vi "Calculate # of Variables per Test.vi"(7 "Seq Parameters":T1={"Test Name"="Unique Test Name", "Target"=enum."cRIO-9012", "Host IP Address"="0.0.0.0", "Target IP Address"="0.0.0.0", "Shared Variable Host"=enum."Target", "Shared Variable Writer"=enum."Target", "Variable Data Type"=enum."Double", "# of Variables per Library"=500, "Update Rate (Hz)"=1.0, "Read Rate (Hz)"=1.0, "Floor"=500, "Ceiling"=5000, "Delta"=500} {"# of Variables per Library" items=["50"=50, "100"=100, "150"=150, "200"=200, "250"=250, "300"=300, "350"=350, "400"=400, "450"=450, "500"=500]; "Delta" min=50 max=1000000 step=50; "Ceiling" min=50 max=1000000 step=50; "Floor" min=50 max=1000000 step=50}, 8 "error in (no error)":errorcluster) -> (0 "error out":errorcluster, 3 "# of Variables per Test":u32[](array[numeric]))   [LabVIEW 2015]
doc: "Create an array that identifies the number of variables needed for each test in the sequence."
uses:
  Type Defs/Sequence Parameters.ctl
  Type Defs/Target Type.ctl
  Type Defs/Variable Data Type.ctl
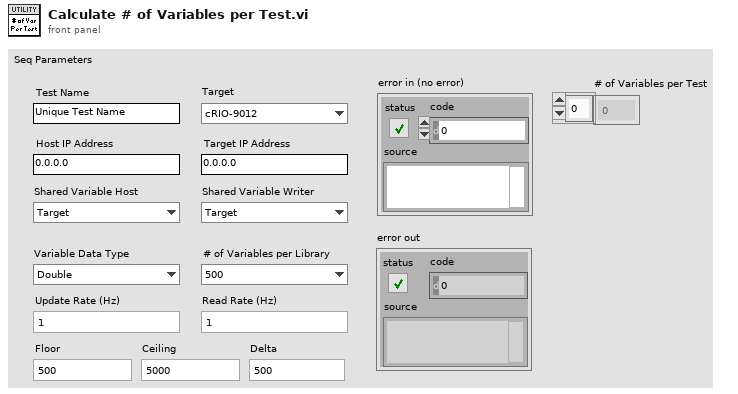
[diagram p1: front panel]
types:
  T1 = typedef "Sequence Parameters.ctl" = cluster{"Test Name":string, "Target":T2, "Host IP Address":string, "Target IP Address":string, "Shared Variable Host":enum16{"Target", "Host"}, "Shared Variable Writer":enum16{"Target", "Host"}, "Variable Data Type":T3, "# of Variables per Library":u16, "Update Rate (Hz)":dbl, "Read Rate (Hz)":dbl, "Floor":u32, "Ceiling":u32, "Delta":u32}
  T2 = typedef "Target Type.ctl" = enum16{"cRIO-9012", "cRIO-9014", "cRIO-9022", "cRIO-9023", "cRIO-9024", "cRIO-9025", "cRIO-9068", "cRIO-9073", "cRIO-9074", "cRIO-9075", "cRIO-9076", "cRIO-9081", "cRIO-9082", "myRIO-1900", "myRIO-1950", "PXI-8101", "PXI-8115", "PXI-8119", "PXI-8820", "PXIe-8100", "PXIe-8101", "PXIe-8133", "PXIe-8135", "PXIe-8820", "sbRIO-9605", "sbRIO-9606", "sbRIO-9623", "sbRIO-9626", "sbRIO-9633", "sbRIO-9636", "Unlisted (Linux-RT)", "Unlisted (PharLap)", "Unlisted (VxWorks)", "Windows Target"}
  T3 = typedef "Variable Data Type.ctl" = enum16{"U8", "U16", "U32", "U64", "I8", "I16", "I32", "I64", "Single", "Double", "Boolean", "String"}
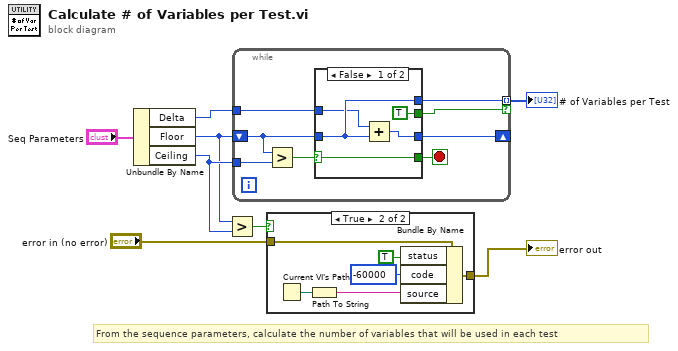
[diagram p0: block diagram]
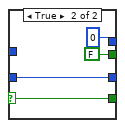
[diagram p3: hidden frame]
diagram:
  # "From the sequence parameters, calculate the number of variables that will be used in each test"
  n1 = Unbundle By Name("Seq Parameters") -> ("Delta"=w7:u32, "Floor"=w4:u32, "Ceiling"=w5:u32)
  n2 = Greater?(x=w4, y=w5) -> (0:w3:bool)
  n3 = while {
    shift-right: [w12] -> _
    shift-left: w4 -> [w15]
    tunnel: [w14] -> w6 mode=indexing if=w11
    tunnel: w7 -> [w13]
    tunnel: w5 -> [w9]
    stop <- w10 stop-if-true
    n4 = Greater?(x=w15, y=w9) -> (0:w16:bool)
    n5 = case shown="False" w16 {
      selector: w16 -> [w17 w22]
      tunnel: w15 -> [w21 w23]
      tunnel: [w21 u32 0 ("Floor")] -> w14
      tunnel: w13 -> [w20 _]
      tunnel: [w19 w23] -> w12
      tunnel: [TRUE FALSE] -> w11
      tunnel: [w17 w22] -> w10
      frame False {
        n6 = Add(x=w20, y=w21) -> (x+y=w19:u32)
      }
      frame True {
      }
    }
  }
  "# of Variables per Test" <- w6
  n7 = case shown="True" w3 {
    tunnel: "error in (no error)" -> [w26 w32]
    tunnel: [w26 w27] -> w1
    frame False {
    }
    frame True {
      n8 = Current VI's Path() -> (path=w29:path)
      n9 = Path To String(path=w29) -> (string=w28:string)
      n10 = Bundle By Name(cluster=w32, "status"=TRUE, "code"=-60000, "source"=w28) -> (w27:errorcluster)
    }
  }
  "error out" <- w1
